vi "Set file permissions on directory files.vi"(7 "Permissions (Writable)":enum16{"Writable", "Read Only"}(ring), 8 "error in (no error)":errorcluster, 11 "Directory":path) -> (0 "error out":errorcluster)   [LabVIEW 2016, in "RT Management.lvlib"]
doc: "Sets the file permissions on every file contained within the provided directory."
uses:
  RT Management.lvlib
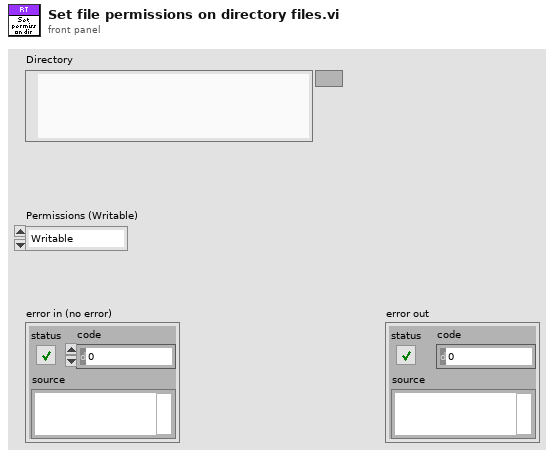
[diagram p1: front panel]
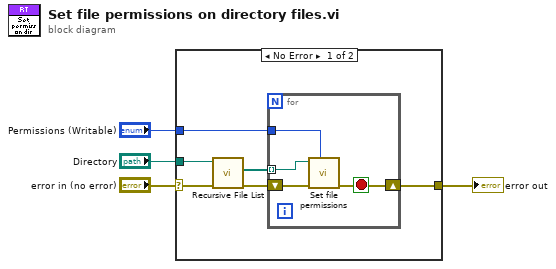
[diagram p0: block diagram]
diagram:
  n1 = case shown="No Error" "error in (no error)" {
    selector: "error in (no error)" -> [w10 w15]
    tunnel: [w5 w15] -> w3
    tunnel: "Directory" -> [w9 _]
    tunnel: "Permissions (Writable)" -> [w6 _]
    frame No Error {
      n2 = call <vilib>:"Recursive File List.vi"("error in (no error)"=w10, "Folder Path"=w9) -> ("error out"=w7:errorcluster, "All Files in Dir"=w8:path[])  [unwired: 5 in, 3 out]
      n3 = for {
        tunnel: w8 -> [w12] mode=indexing
        tunnel: w6 -> [w13]
        shift-right: [w11] -> w5
        shift-left: w7 -> [w14]
        stop <- w11 stop-if-true
        n4 = call "Set file permissions.vi"("Permissions (Writable)"=w13, "error in"=w14, "Path"=w12) -> ("error out"=w11:errorcluster)  [unwired: 7 in, 1 out]
      }
    }
    frame Error {
    }
  }
  "error out" <- w3
